vi "test.vi"   [LabVIEW 2024]
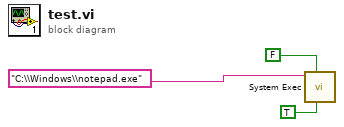
[diagram p0: block diagram]
diagram:
  n1 = call <vilib>:"System Exec.vi"("run minimized? (F)"=TRUE, "wait until completion? (T)"=FALSE, "command line"="C:\\Windows\\notepad.exe") -> ()  [unwired: 5 in, 4 out]
